vi "Initialise Generic Actor.vi"(4 "Sub Panel":refnum<vi>, 6 "Name":string, 7 "Close FP On Shutdown (T)":bool=TRUE, 8 "error in (no error)":errorcluster, 9 "Front Panel State":T1=enum."Standard", 10 "Response Channel":refnum<class "Messenger.lvclass">, 11 "Actor in":refnum<class "Actor.lvclass">) -> (0 "error out":errorcluster, 3 "Actor out":refnum<class "Actor.lvclass">)   [LabVIEW 2015, in "Actor.lvclass"]
doc: "<b>Response</b> channel is used by this actor to return infomation back to the parent."
uses:
  Actor.lvclass
  Messaging/Messenger/Messenger.lvclass
  Front Panel State.ctl
  Actor.lvclass/Actor.ctl
  Utility/Utility.lvlib
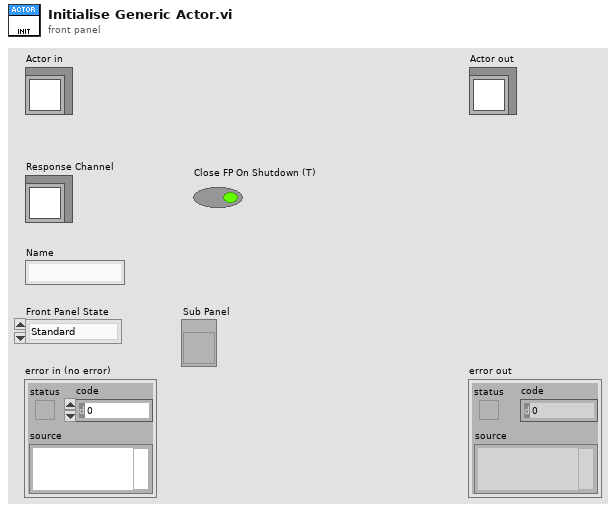
[diagram p1: front panel]
types:
  T1 = typedef "Actor.lvclass/Front Panel State.ctl" = enum32{"Invalid", "Standard", "Closed", "Hidden", "Minimized", "Maximized"}
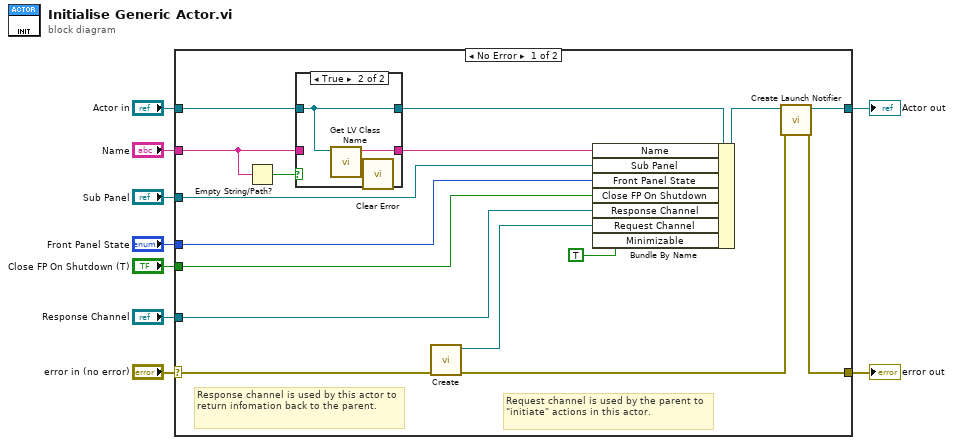
[diagram p0: block diagram]
diagram:
  n1 = case shown="No Error" "error in (no error)" {
    selector: "error in (no error)" -> [w25 w32]
    tunnel: [w11 w32] -> w8
    tunnel: [w13 w31] -> w1
    tunnel: "Actor in" -> [w22 w31]
    tunnel: "Response Channel" -> [w18 _]
    tunnel: "Name" -> [w23 _]
    tunnel: "Front Panel State" -> [w20 _]
    tunnel: "Close FP On Shutdown (T)" -> [w19 _]
    tunnel: "Sub Panel" -> [w15 _]
    frame No Error {
      # "Response channel is used by this actor to return infomation back to the parent."
      # "Request channel is used by the parent to \"initiate\" actions in this actor."
      n2 = Empty String/Path?(string/path=w23) -> (empty?=w24:bool)
      n3 = case shown="True" w24 {
        tunnel: w23 -> [w27 _]
        tunnel: [w27 w29] -> w16
        tunnel: w22 -> [w26 w30]
        tunnel: [w26 w30] -> w21
        frame False {
        }
        frame True {
          n4 = call <vilib>:"Get LV Class Name.vi"("object"=w30) -> ("error out"=w28:errorcluster, "class name"=w29:string)  [unwired: 9 in]
          n5 = call "Clear Error.vi"("error in (no error)"=w28) -> ()  [unwired: 1 out]
        }
      }
      n6 = call "Create.vi"("error in (no error)"=w25) -> ("error out"=w12:errorcluster, "Messenger out"=w17:refnum<class "Messenger.lvclass">)  [unwired: 9 in]
      n7 = Bundle By Name(cluster=w21, "Name"=w16, "Sub Panel"=w15, "Front Panel State"=w20, "Close FP On Shutdown"=w19, "Response Channel"=w18, "Request Channel"=w17, "Minimizable"=TRUE) -> (w14:refnum<class "Actor.lvclass">)
      n8 = call-dynamic "Create Launch Notifier.vi"("error in (no error)"=w12, "Actor in"=w14) -> ("error out"=w11:errorcluster, "Actor out"=w13:refnum<class "Actor.lvclass">)  [unwired: 8 in]
    }
    frame Error {
    }
  }
  "error out" <- w8
  "Actor out" <- w1
